vi "Digital.vi"(0 "Delimiter":string="\t", 1 "Data":string) -> ()   [LabVIEW 2014]
uses:
  <vilib>/Waveform/DTblOps.llb/DTbl Spreadsheet String to Digital.vi
panel:
  out "Digital Waveform Graph":digitaldata(graph)
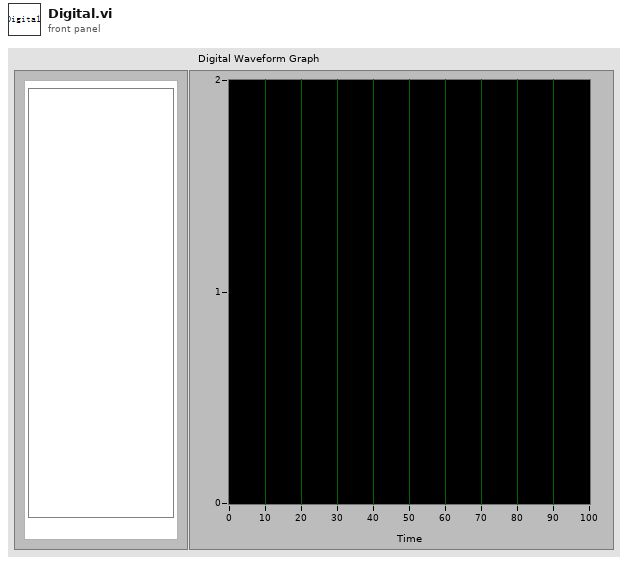
[diagram p1: front panel]
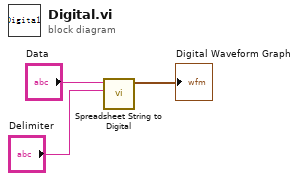
[diagram p0: block diagram]
diagram:
  n1 = call-poly <vilib>:"Spreadsheet String to Digital.vi"("delimiter (tab)"="Delimiter", "spreadsheet string"="Data") -> ("digital data"=→"Digital Waveform Graph":digitaldata)  [unwired: 8 in, 1 out]
